vi "PH_Timing.Set GateGen on Mode Change.vi"(0 "i ref in":refnum<vi>, 5 "error in (no error)":errorcluster) -> (14 "i ref out":refnum<vi>, 19 "error out":errorcluster)   [LabVIEW 2014, in "PH_Timing.lvlib"]
doc: "This VI sets changes in case of a timing mode change to the GateGen Gater GD. This is relevant actually only if it changed from Shotmode to a non Shotmode or the other way round."
uses:
  PH_Timing.lvlib
  CS_DigitalIO/BNC555/BNC555.lvlib
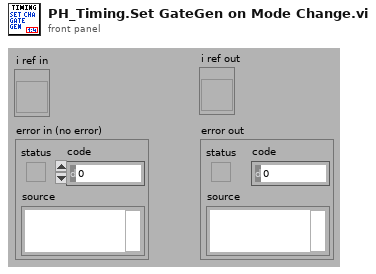
[diagram p1: front panel]
types:
  T1 = enum16{"Normal", "Single", "Burst", "Duty Cycle"}
  T2 = enum16{"Normal", "Single", "Burst", "Divide by N"}
  T3 = typedef "PH_Timing.lvlib/PH_Timing.i attribute.ctl" = cluster{"Sequencer":cluster{"linked?":bool, "Proc State":string, "Ref State":refnum<vi>}, "Gate Generator":cluster{"GD":cluster{"Device Status":T4, "linked?":bool}, "Settings":T5, "GUI Ref":refnum<vi>}, "Interlock Bypass":cluster{"Instancename":string, "Switch linked?":bool, "Device Status":T4, "Ref Status":refnum<vi>}, "Roughtuner":cluster{"Settings":T6, "GUI Ref":refnum<vi>, "GD":cluster{"Device Status":T4, "linked?":bool}}, "0,5Hz Gater":cluster{"Settings":T7, "GUI Ref":refnum<vi>, "GD":cluster{"Device Status":T4, "linked?":bool}}, "Slow Trigger":cluster{"Settings":T8, "GUI Ref":refnum<vi>, "Service ID Delay":i32, "Service ID Ext Trig":i32, "Wanted Settings":T8}, "Timing Mode":cluster{"Mode":T9, "GUI Ref":refnum<vi>, "Service ID T2":i32, "Service ID Mode":i32, "Wanted Mode":T9}, "ns Generator":cluster{"Settings":T10, "ns Generator Settings":refnum<vi>, "GD":cluster{"Device Status":T4, "linked?":bool}}, "Phase FEs":cluster{"Settings":T13, "GUI Ref":refnum<vi>, "Service ID Phase":i32, "Wanted Settings":T13}, "GD GUI Refs":refnum<vi>[], "Heads":T14[], "GUI Ref Delete":refnum<vi>}
  T4 = typedef "PH_StatusHandler.lvlib/PH_StatusHandler.Status.ctl" = i16
  T5 = typedef "PH_Timing.lvlib/PH_Timing.GateGen.ctl" = cluster{"Instance":string, "Channel Gate":i32, "Channel T2":i32, "Width Gate":dbl, "Width T2":dbl, "Delay Gate":dbl, "Delay T2":dbl, "Gate activ":bool, "T2 activ":bool, "System Mode":enum16{"Normal", "Single", "Burst", "Duty Cycle"}}
  T6 = typedef "PH_Timing.lvlib/PH_Timing.Roughtuner.ctl" = cluster{"Instance":string, "Phase PHELIX / UNILAC":cluster{"Channel":u16, "relative to":u16, "Delay [ms]":dbl}, "Pulse Length":cluster{"Channel":u16, "relative to":u16, "Delay [ms]":dbl}, "Trigger":cluster{"externally?":bool, "Rate [Hz]":dbl}}
  T7 = typedef "PH_Timing.lvlib/PH_Timing.0.5HzGater.ctl" = cluster{"Instance":string, "Channel ns FE Delay":i32, "Channel 0.5Hz":i32, "Width ns FE Delay":dbl, "Width 0.5Hz":dbl, "Delay ns FE Delay":dbl, "Delay 0.5Hz":dbl, "ns FE Delay active":bool, "0.5Hz activ":bool, "ns FE Delay inverted":bool, "0.5Hz inverted":bool}
  T8 = typedef "PH_Timing.lvlib/PH_Timing.Slow Trigger Settings.ctl" = cluster{"Delay":dbl, "externally triggered?":bool}
  T9 = typedef "PH_Timing.lvlib/PH_Timing.Timing Mode.ctl" = cluster{"T2":i16, "Modeselector":enum32{"10 Hz", "0.5 Hz", "Shot"}}
  T10 = typedef "PH_Timing.lvlib/PH_Timing.ns Generator.ctl" = cluster{"Instance":string, "Phase fs / ns FE":cluster{"Channel":T11, "Settings":T12}}
  T11 = typedef "Stanford Research DG645 - Driver.lvlib/Channel.ctl" = i32
  T12 = typedef "PH_SRDG645.lvlib/PH_SRDG645.Channel Settings.ctl" = cluster{"Delay [s]":dbl, "relative to":i32}
  T13 = typedef "PH_Timing.lvlib/PH_Timing.Phase FEs.ctl" = cluster{"Phase":dbl}
  T14 = typedef "PH_Timing.lvlib/PH_Timing.PU Data.ctl" = cluster{"linked?":bool, "Data":T15, "GD":cluster{"Device Status":T4, "linked?":bool}, "GUI Ref":refnum<vi>, "PU":T16}
  T15 = typedef "PH_Timing.lvlib/PH_Timing.PU Info.ctl" = cluster{"Act CH?":bool, "GD":string, "CH":i32, "Delay":dbl, "active":bool, "in Use?":bool}
  T16 = typedef "PH_PP_Common.lvlib/PH_PP_Common.PUs.ctl" = enum16{"no Info", "PA-19mm-1", "PA-19mm-2", "PA-45mm-PILC", "PA-45mm-MAIN", "MA-PU-1", "MA-PU-2", "MA-PU-3", "MA-PU-4", "MA-PU-5", "MA-PU-6", "MA-FR", "MA-PILC", "PA-45mm-DP"}
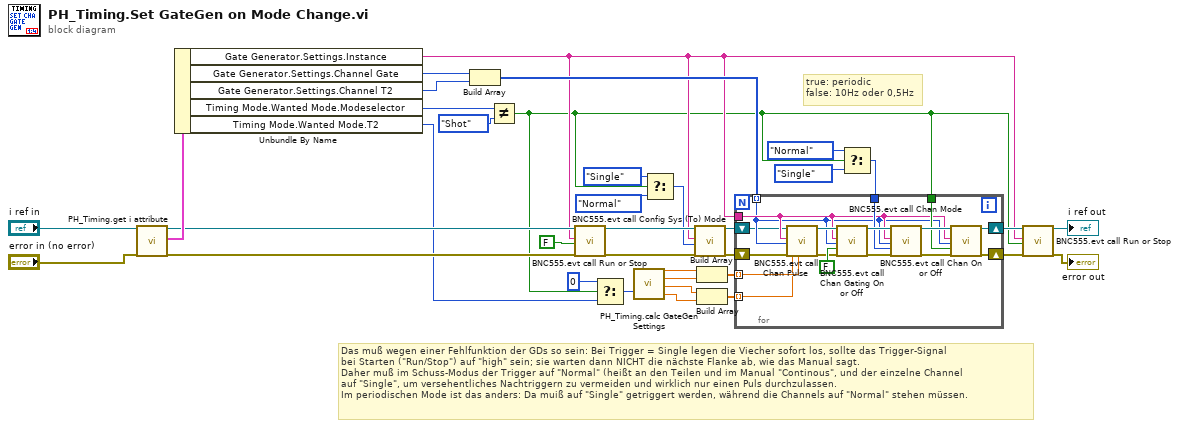
[diagram p0: block diagram]
diagram:
  # "true: periodic\nfalse: 10Hz oder 0,5Hz"
  # "Das muß wegen einer Fehlfunktion der GDs so sein: Bei Trigger = Single legen die Viecher sofort los, sollte das Trigger-Signal \nbei Starten (\"Run/Stop\") auf \"high\" sein; sie warten dann NICHT die nächste Flanke ab, wie das Manual sagt.\nDaher muß im Schuss-Modus der Trigger auf \"Normal\" (heißt an den Teilen und im Manual \"Continous\", und der einzelne Channel\nauf \"Single\", um versehentliches Nachtriggern zu vermeiden und wirklich nur einen Puls durchzulassen.\nIm periodischen Mode ist das anders: Da muiß auf \"Single\" getriggert werden, während die Channels auf \"Normal\" stehen müssen."
  n1 = call "PH_Timing.get i attribute.vi"("i ref in"="i ref in", "error in (no error)"="error in (no error)") -> ("i ref out"=w30:refnum<vi>, "i attribute"=w34:T3, "error out"=w31:errorcluster)  [unwired: 15 in]
  n2 = Unbundle By Name(w34) -> ("Gate Generator.Settings.Instance"=w7:string, "Gate Generator.Settings.Channel Gate"=w33:i32, "Gate Generator.Settings.Channel T2"=w32:i32, "Timing Mode.Wanted Mode.Modeselector"=w24:enum32{"10 Hz", "0.5 Hz", "Shot"}, "Timing Mode.Wanted Mode.T2"=w4:i16)
  n3 = Build Array(w33, w32) -> (w29:i32[])
  n4 = Not Equal?(x=w24, y=enum32{"10 Hz", "0.5 Hz", "Shot"}."Shot" ("Timing Mode.Mode.Modeselector")) -> (x != y?=w3:bool)
  n5 = call "BNC555.evt call Run or Stop.vi"("i ref in"=w30, "Generator Instance"=w7, "Start\\Stop"=FALSE ("Start\\Stop"), "error in (no error)"=w31) -> ("i ref out"=w13:refnum<vi>, "error out"=w12:errorcluster)  [unwired: 14 in]
  n6 = Select(t=i16 0, s=w3, f=w4) -> (s? t:f=w5:i16)
  n7 = call "PH_Timing.calc GateGen Settings.vi"("T2 [s]"=w5) -> ("Width Gate"=w22:dbl, "Width T2"=w21:dbl, "Delay Gate"=w20:dbl, "Delay T2"=w19:dbl)  [unwired: 23 in]
  n8 = Select(t=T1."Single" ("Mode"), s=w3, f=T1."Normal" ("Mode")) -> (s? t:f=w8:T1)
  n9 = call "BNC555.evt call Config Sys (To) Mode.vi"("i ref in"=w13, "Generator Instance"=w7, "Mode"=w8, "error in (no error)"=w12) -> ("i ref out"=w2:refnum<vi>, "error out"=w1:errorcluster)  [unwired: 14 in]
  n10 = Build Array(w22, w21) -> (w27:dbl[])
  n11 = Build Array(w20, w19) -> (w28:dbl[])
  n12 = Select(t=T2."Normal" ("Mode (0:Normal)"), s=w3, f=T2."Single" ("Mode (0:Normal)")) -> (s? t:f=w17:T2)
  n13 = for {
    shift-right: [w46] -> w16
    shift-left: w2 -> [w38]
    shift-right: [w48] -> w15
    shift-left: w1 -> [w37]
    tunnel: w7 -> [w40]
    tunnel: w29 -> [w39] mode=indexing
    tunnel: w27 -> [w42] mode=indexing
    tunnel: w28 -> [w41] mode=indexing
    tunnel: w17 -> [w50]
    tunnel: w3 -> [w45]
    n14 = call "BNC555.evt call Chan Pulse.vi"("i ref in"=w38, "Generator Instance"=w40, "Channel"=w39, "error in (no error)"=w37, "Delay"=w41, "Width"=w42) -> ("i ref out"=w44:refnum<vi>, "error out"=w43:errorcluster)  [unwired: 12 in]
    n15 = call "BNC555.evt call Chan Gating On or Off.vi"("i ref in"=w44, "Generator Instance"=w40, "Channel"=w39, "Gating State"=FALSE ("Gate enabled (false)"), "error in (no error)"=w43) -> ("i ref out"=w51:refnum<vi>, "error out"=w52:errorcluster)  [unwired: 13 in]
    n16 = call "BNC555.evt call Chan Mode.vi"("i ref in"=w51, "Generator Instance"=w40, "Channel"=w39, "Mode"=w50, "error in (no error)"=w52) -> ("i ref out"=w47:refnum<vi>, "error out"=w49:errorcluster)  [unwired: 13 in]
    n17 = call "BNC555.evt call Chan On or Off.vi"("i ref in"=w47, "Generator Instance"=w40, "Channel"=w39, "State"=w45, "error in (no error)"=w49) -> ("i ref out"=w46:refnum<vi>, "error out"=w48:errorcluster)  [unwired: 13 in]
  }
  n18 = call "BNC555.evt call Run or Stop.vi"("i ref in"=w16, "Generator Instance"=w7, "Start\\Stop"=w3, "error in (no error)"=w15) -> ("i ref out"=→"i ref out":refnum<vi>, "error out"=→"error out":errorcluster)  [unwired: 14 in]
